vi "15_1.vi"() -> ()   [LabVIEW 2018]
panel:
  in  "Turn":i32=2020
  out "element":i32=232
  out "Array":i32[](array[numeric])=[2, 1, 10, 11, 0, 6, 0, 2, 7, 0, 3, 0, 2, 5, 0, 3, 5, 3, 2, 6, 14, 0, 7, 14, 3, 7, 3, 2, 9, 0, 8, 0, 2, 5, 17, 0, 4, 0, 2, 6, 20, 0, 4, 6, 4, 2, 7, 21, 0, 7, 3, 24, 0, 4, 9, 26, 0, 4, 4, 1, 58, 0, 5, 29, 0, 3, 15, 0, 3, 3, 1, 11, 68, 0, 6, 31, 0, 3, 8, 48, 0, 4, 23, 0, 3, 7, 36, 0, 4, 7, 4, 2, 46, 0, 6, 20, 55, 0, 4, 8, 21, 53, 0, 5, 41, 0, 3, 22, 0, 3, 3, 1, 41, 8, 14, 91, 0, 8, 4, 20, 24, 69, 0, 6, 29, 61, 0, 4, 9, 74, 0, 4, 4, 1, 22, 27, 0, 6, 14, 24, 19, 0, 5, 39, 0, 3, 35, 0, 3, 3, 1, 17, 117, 0, 6, 17, 4, 24, 18, 0, 6, 6, 1, 12, 0, 5, 23, 84, 0, 4, 13, 0, 3, 23, 7, 85, 0, 5, 12, 15, 113, 0, 5, 5, 1, 22, 51, 0, 6, 27, 54, 0, 4, 23, 20, 75, 0, 5, 14, 60, 0, 4, 9, 74, 74, 1, 21, 106, 0, 8, 92, 0, 3, 40, 0, 3, 3, 1, 12, 40, 6, 32, 0, 8, 14, 26, 170, 0, 5, 31, 154, 0, 4, 31, 4, 2, 144, 0, 6, 18, 81, 0, 4, 8, 20, 50, 0, 5, 19, 108, 0, 4, 9, 50, 8, 11, 184, 0, 7, 84, 92, 50, 8, 8, 1, 47, 0, 9, 15, 89, 0, 4, 20, 28, 0, 4, 4, 1, 13, 108, 30, 0, 7, 24, 126, 0, 4, 10, 285, 0, 4, 4, 1, 15, 25, 0, 6, 58, 237, 0, 4, 9, 34, 0, 4, 4, 1, 14, 83, 0, 6, 14, 4, 7, 31, 81, 75, 121, 0, 9, 18, 81, 6, 12, 105, 0, 7, 13, 49, 0, 4, 18, 11, 77, 0, 5, 88, 0, 3, 122, 0, 3, 3, 1, 37, 0, 5, 11, 15, 55, 253, 0, 6, 30, 73, 0, 4, 26, 132, 0, 4, 4, 1, 19, 115, 0, 6, 14, 56, 0, 4, 9, 52, 0, 4, 4, 1, 14, 10, 91, 264, 0, 8, 119, 0, 3, 43, 0, 3, 3, 1, 14, 14, 1, 3, 5, 49, 68, 325, 0, 12, 77, 68, 5, 8, 22, 220, 0, 8, 4, 34, 108, 132, 54, 223, 0, 8, 8, 1, 25, 125, 0, 6, 56, 55, 75, 109, 0, 6, 6, 1, 12, 31, 118, 0, 7, 109, 10, 59, 0, 5, 37, 97, 0, 4, 35, 299, 0, 4, 4, 1, 20, 179, 0, 6, 25, 36, 370, 0, 5, 19, 97, 19, 2, 228, 0, 7, 31, 35, 23, 276, 0, 6, 18, 142, 0, 4, 27, 288, 0, 4, 4, 1, 32, 262, 0, 6, 14, 95, 0, 4, 9, 120, 0, 4, 4, 1, 14, 10, 61, 374, 0, 8, 85, 328, 0, 4, 11, 160, 0, 4, 4, 1, 16, 0, 5, 56, 93, 0, 4, 8, 18, 48, 443, 0, 6, 39, 383, 0, 4, 10, 32, 48, 10, 3, 140, 0, 8, 17, 383, 12, 109, 105, 218, 0, 8, 8, 1, 35, 80, 0, 6, 26, 195, 0, 4, 26, 4, 2, 95, 71, 0, 7, 96, 0, 3, 31, 99, 0, 4, 12, 30, 218, 29, 449, 0, 7, 14, 80, 29, 6, 29, 2, 24, 300, 0, 10, 53, 486, 0, 4, 21, 385, 0, 4, 4, 1, 49, 201, 0, 6, 20, 150, 0, 4, 9, 114, 0, 4, 4, 1, 14, 34, 202, 0, 7, 39, 90, 0, 4, 10, 34, 9, 17, 85, 121, 308, 0, 9, 6, 29, 49, 34, 11, 126, 350, 0, 9, 9, 1, 29, 10, 21, 51, 457, 0, 9, 8, 101, 0, 4, 31, 85, 28, 380, 0, 6, 27, 180, 0, 4, 10, 20, 61, 164, 0, 6, 10, 6, 2, 87, 0, 6, 4, 13, 347, 0, 5, 162, 0, 3, 115, 317, 0, 4, 11, 52, 314, 0, 5, 12, 120, 199, 0, 5, 5, 1, 57, 0, 5, 4, 16, 188, 0, 5, 5, 1, 10, 40, 489, 0, 7, 96, 149, 0, 4, 15, 368, 0, 4, 4, 1, 15, 6, 51, 81, 404, 0, 9, 82, 0, 3, 51, 8, 86, 0, 5, 31, 86, 4, 19, 278, 0, 7, 32, 213, 0, 4, 8, 15, 27, 93, 234, 0, 7, 11, 70, 0, 4, 11, 4, 2, 92, 502, 0, 7, 11, 7, 2, 7, 2, 2, 1, 51, 41, 662, 0, 12, 87, 108, 368, 63, 0, 6, 60, 585, 0, 4, 27, 38, 0, 4, 4, 1, 21, 152, 0, 6, 14, 187, 0, 4, 9, 74, 599, 0, 5, 70, 51, 35, 261, 0, 6, 15, 64, 0, 4, 15, 4, 2, 48, 288, 343, 0, 8, 76, 0, 3, 96, 116, 0, 4, 13, 158, 0, 4, 4, 1, 44, 0, 5, 34, 209, 0, 4, 8, 21, 52, 161, 0, 6, 38, 62, 0, 4, 10, 148, 0, 4, 4, 1, 23, 392, 0, 6, 14, 67, 0, 4, 9, 67, 4, 3, 45, 0, 7, 106, 669, 0, 4, 8, 35, 72, 0, 5, 44, 47, 621, 0, 5, 5, 1, 31, 155, 0, 6, 31, 4, 18, 377, 0, 6, 6, 1, 12, 127, 0, 6, 5, 18, 11, 144, 675, 0, 7, 39, 299, 470, 0, 5, 11, 10, 66, 0, 5, 5, 1, 23, 66, 6, 22, 525, 0, 9, 64, 120, 244, 0, 5, 13, 107, 0, 4, 45, 70, 137, 0, 5, 9, 15, 132, 538, 0, 6, 24, 371, 0, 4, 15, 9, 11, 40, 253, 612, 0, 8, 85, 314, 280, 0, 5, 23, 44, 87, 195, 421, 0, 7, 63, 197, 0, 4, 24, 28, 330, 0, 5, 16, 286, 0, 4, 9, 32, 248, 0, 5, 9, 5, 2, 179, 547, 0, 7, 25, 548, 0, 4, 16, 20, 346, 0, 5, 14, 147, 0, 4, 9, 20, 9, 2, 21, 174, 0, 8, 58, 727, 0, 4, 12, 124, 0, 4, 4, 1, 107, 94, 0, 6, 84, 779, 0, 4, 9, 24, 61, 381, 0, 6, 10, 127, 144, 139, 0, 6, 6, 1, 22, 126, 423, 0, 7, 58, 37, 621, 176, 0, 6, 12, 39, 153, 0, 5, 60, 288, 252, 0, 5, 5, 1, 23, 108, 301, 0, 7, 23, 5, 8, 63, 109, 547, 89, 821, 0, 10, 45, 151, 0, 4, 56, 582, 0, 4, 4, 1, 25, 101, 457, 462, 0, 8, 23, 26, 555, 0, 5, 29, 475, 0, 4, 16, 112, 0, 4, 4, 1, 21, 105, 584, 0, 7, 46, 1038, 0, 4, 10, 41, 361, 0, 5, 24, 96, 312, 0, 5, 5, 1, 21, 21, 1, 3, 277, 0, 9, 110, 0, 3, 6, 90, 540, 0, 5, 16, 42, 0, 4, 31, 269, 0, 4, 4, 1, 22, 115, 491, 0, 7, 46, 46, 1, 8, 70, 236, 0, 8, 4, 15, 227, 0, 5, 28, 206, 0, 4, 8, 10, 60, 123, 0, 6, 42, 37, 138, 0, 5, 15, 19, 465, 0, 5, 5, 1, 32, 219, 0, 6, 16, 54, 803, 0, 5, 10, 26, 110, 69, 1102, 0, 7, 51, 419, 0, 4, 38, 380, 578, 0, 5, 16, 21, 90, 81, 514, 0, 7, 16, 7, 2, 226, 0, 6, 34, 408, 0, 4, 22, 82, 525, 324, 0, 6, 10, 39, 192, 0, 5, 28, 75, 840, 0, 5, 5, 1, 60, 76, 447, 0, 7, 31, 111, 0, 4, 27, 492, 0, 4, 4, 1, 15, 82, 33, 0, 7, 15, 5, 23, 183, 0, 6, 38, 66, 370, 842, 0, 6, 6, 1, 19, 100, 0, 6, 5, 17, 687, 0, 5, 4, 30, 744, 0, 5, 5, 1, 16, 78, 0, 6, 16, 4, 12, 260, 0, 6, 6, 1, 12, 6, 3, 180, 678, 0, 9, 187, 541, 0, 4, 17, 34, 96, 206, 157, 0, 7, 60, 80, 774, 0, 5, 36, 900, 0, 4, 16, 35, 480, 0, 5, 9, 26, 145, 0, 5, 5, 1, 39, 112, 253, 412, 0, 8, 184, 1122, 0, 4, 22, 129, 0, 4, 4, 1, 16, 28, 125, 970, 0, 8, 16, 6, 61, 352, 0, 6, 4, 14, 389, 0, 5, 34, 60, 55, 983, 0, 6, 11, 451, 0, 4, 14, 14, 1, 30, 103, 0, 7, 71, 862, 0, 4, 11, 15, 136, 0, 5, 26, 65, 0, 4, 9, 70, 256, 0, 5, 9, 5, 2, 197, 464, 0, 7, 25, 343, 626, 0, 5, 10, 193, 0, 4, 21, 219, 245, 0, 5, 9, 21, 6, 53, 877, 0, 7, 21, 6, 6, 1, 54, 256, 36, 118, 1042, 0, 11, 52, 632, 0, 4, 27, 203, 0, 4, 4, 1, 17, 145, 123, 295, 0, 8, 101, 390, 0, 4, 11, 21, 32, 290, 0, 6, 34, 100, 200, 0, 5, 49, 879, 0, 4, 15, 87, 542, 0, 5, 9, 58, 459, 0, 5, 5, 1, 37, 326, 0, 6, 25, 83, 1223, 0, 5, 10, 83, 5, 3, 203, 55, 133, 0, 9, 24, 405, 0, 4, 34, 43, 1163, 0, 5, 15, 39, 182, 0, 5, 5, 1, 34, 12, 228, 1098, 0, 8, 71, 144, 517, 0, 5, 12, 10, 37, 47, 688, 0, 7, 110, 356, 0, 4, 34, 22, 201, 986, 0, 6, 58, 68, 1187, 0, 5, 22, 10, 22, 2, 154, 1367, 0, 8, 35, 240, 0, 4, 23, 312, 465, 401, 0, 6, 23, 6, 2, 17, 125, 225, 0, 8, 18, 710, 0, 4, 18, 4, 2, 12, 55, 87, 113, 1449, 0, 10, 38, 336, 0, 4, 12, 11, 139, 588, 0, 6, 30, 225, 28, 256, 173, 0, 7, 72, 768, 0, 4, 17, 40, 694, 0, 5, 66, 361, 524, 0, 5, 5, 1, 106, 790, 0, 6, 27, 187, 331, 0, 5, 10, 43, 127, 628, 0, 6, 11, 43, 6, 3, 146, 0, 7, 38, 55, 62, 838, 0, 6, 10, 19, 390, 200, 190, 0, 7, 13, 762, 0, 4, 51, 478, 0, 4, 4, 1, 45, 617, 0, 6, 21, 215, 0, 4, 9, 176, 656, 0, 5, 49, 214, 0, 4, 9, 9, 1, 20, 714, 0, 7, 34, 153, 667, 0, 5, 16, 346, 732, 0, 5, 5, 1, 16, 7, 14, 333, 0, 8, 134, 0, 3, 71, 190, 59, 1320, 0, 6, 47, 188, 1061, 0, 5, 21, 52, 289, 0, 5, 5, 1, 27, 104, 0, 6, 16, 31, 503, 0, 5, 10, 89, 694, 129, 403, 0, 7, 41, 655, 0, 4, 66, 135, 0, 4, 4, 1, 26, 369, 0, 6, 26, 4, 7, 17, 153, 72, 159, 0, 9, 83, 277, 664, 0, 5, 35, 217, 0, 4, 16, 44, 851, 0, 5, 9, 15, 275, 0, 5, 5, 1, 34, 99, 1268, 0, 7, 32, 338, 0, 4, 21, 76, 572, 0, 5, 15, 20, 118, 375, 0, 6, 50, 1593, 0, 4, 15, 10, 76, 16, 39, 308, 1237, 0, 9, 39, 5, 21, 26, 66, 77, 1471, 0, 9, 9, 1, 44, 55, 190, 123, 390, 186, 0, 10, 26, 16, 26, 2, 264, 1510, 0, 8, 141, 0, 3, 141, 3, 2, 10, 15, 43, 220, 1497, 0, 10, 6, 54, 436, 0, 5, 43, 10, 7, 76, 55, 37, 344, 0, 9, 44, 43, 10, 10, 1, 48, 1106, 0, 9, 9, 1, 6, 25, 403, 147, 922, 0, 9, 8, 46, 763, 0, 5, 32, 105, 819, 0, 5, 5, 1, 19, 256, 306, 0, 7, 41, 166, 0, 4, 102, 0, 3, 64, 1029, 0, 4, 7, 12, 331, 297, 0, 6, 40, 318, 0, 4, 10, 53, 514, 739, 0, 6, 10, 6, 2, 86, 1248, 0, 7, 22, 395, 0, 4, 17, 187, 324, 740, 0, 6, 15, 99, 166, 45, 292, 0, 7, 17, 13, 307, 0, 5, 62, 322, 0, 4, 22, 26, 129, 232]
  in  "Input":string="2,1,10,11,0,6"
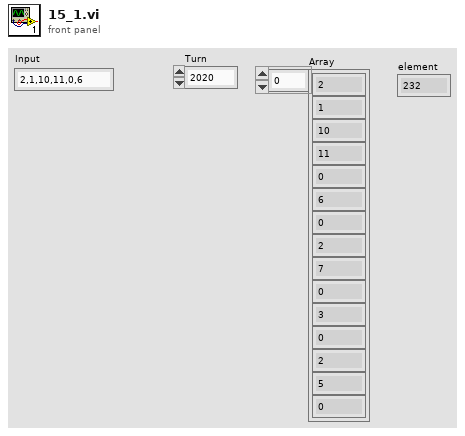
[diagram p1: front panel]
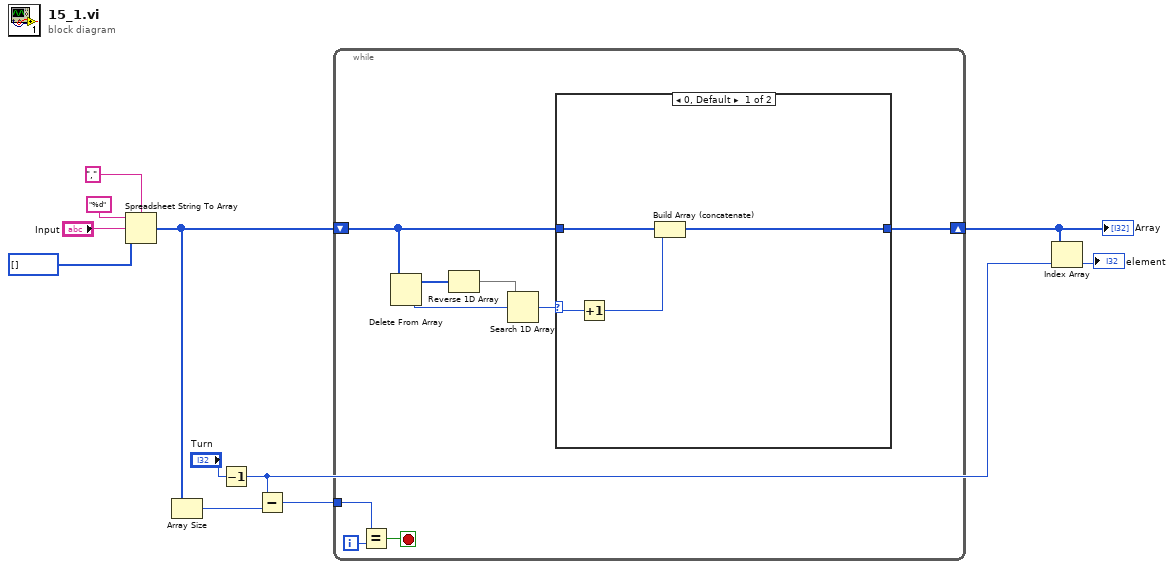
[diagram p0: block diagram]
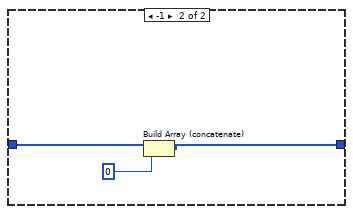
[diagram p2: hidden frame]
diagram:
  n1 = Spreadsheet String To Array(delimiter (Tab)=",", format string="%d", spreadsheet string="Input", array type (2D Dbl)=i32[] []) -> (array=w7:i32[])
  n2 = Array Size(array=w7) -> (size(s)=w6:i32)
  n3 = Decrement(x="Turn") -> (x-1=w1:i32)
  n4 = Subtract(x=w1, y=w6) -> (x-y=w3:i32)
  n5 = while {
    shift-right: [w19] -> w5
    shift-left: w7 -> [w15]
    tunnel: w3 -> [w17]
    i -> [w18]
    stop <- w16 stop-if-true
    n6 = Equal?(x=w17, y=w18) -> (x = y?=w16:bool)
    n7 = Delete From Array(array=w15) -> (deleted portion=w14:i32, array with subset deleted=w13:i32[])  [unwired: 2 in]
    n8 = Reverse 1D Array(array=w13) -> (reversed array=w12:i32[])
    n9 = Search 1D Array(1D array=w12, element=w14) -> (index of element=w20:i32)  [unwired: 1 in]
    n10 = case shown="0, Default" w20 {
      selector: w20 -> [w24 _]
      tunnel: w15 -> [w23 w27]
      tunnel: [w21 w25] -> w19
      frame 0, Default {
        n11 = Increment(x=w24) -> (x+1=w22:i32)
        n12 = Build Array (concatenate)(w23, w22) -> (w21:i32[])
      }
      frame -1 {
        n13 = Build Array (concatenate)(w27, 0) -> (w25:i32[])
      }
    }
  }
  "Array" <- w5
  n14 = Index Array(array=w5, index=w1) -> (element=→"element":i32)
